vi "getWindowSnapshot.vi"(8 "error in (no error)":errorcluster, 11 "Registered Name":string) -> (0 "error out":errorcluster, 3 "Cropped Image Data":T1)   [LabVIEW 2018, in "Image_Diff.lvlib"]
uses:
  Image_Diff.lvlib
  <vilib>/picture/picture.llb/imagedata.ctl
panel:
  out "Cropped Picture":picture
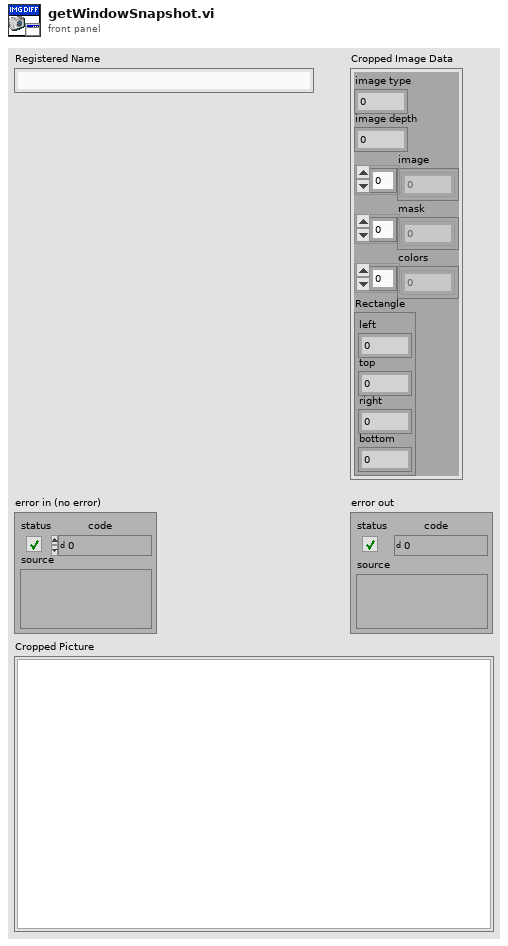
[diagram p1: front panel]
types:
  T1 = typedef "imagedata.ctl" = cluster{"image type":i32, "image depth":i32, "image":u8[], "mask":u8[], "colors":u32[], "Rectangle":cluster{"left":i16, "top":i16, "right":i16, "bottom":i16}}
  T2 = cluster{"left":i32, "top":i32, "right":i32, "bottom":i32}
  T3 = enum32{"Invalid", "Standard", "Closed", "Hidden", "Minimized", "Maximized"}
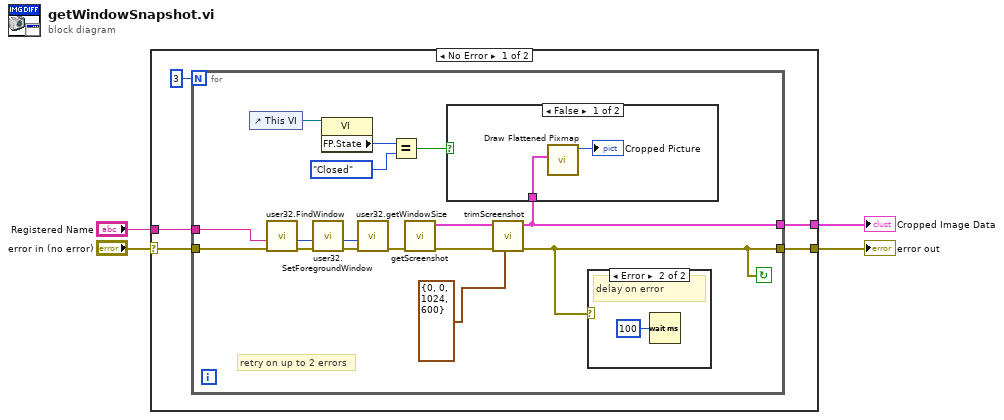
[diagram p0: block diagram]
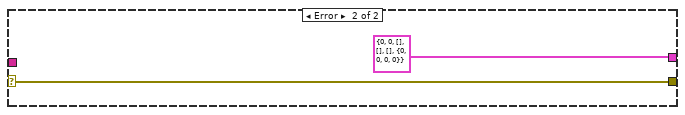
[diagram p4: hidden frame]
diagram:
  n1 = case shown="No Error" "error in (no error)" {
    selector: "error in (no error)" -> [w9 w29]
    tunnel: "Registered Name" -> [w6 _]
    tunnel: [w8 w29] -> w2
    tunnel: [w7 T1 {"image type"=0, "image depth"=0, "image"=[], "mask"=[], "colors"=[], "Rectangle"={"left"=0, "top"=0, "right"=0, "bottom"=0}} ("Cropped Image Data")] -> w1
    frame No Error {
      n2 = for {
        N: 3 -> [_]
        tunnel: [w13] -> w7
        tunnel: w6 -> [w12]
        tunnel: w9 -> [w21]
        tunnel: [w10] -> w8
        stop <- w10 continue-if-true
        # "retry on up to 2 errors"
        n3 = control-ref of="This VI"() -> (w17:refnum<vi>)
        n4 = call "user32.FindWindow.vi"("error in"=w21, "Window Title"=w12) -> ("error out"=w25:errorcluster, "hWnd"=w23:u32)  [unwired: 8 in]
        n5 = call "user32.SetForegroundWindow.vi"("error in"=w25, "hWnd"=w23) -> ("error out"=w24:errorcluster, "hWnd out"=w22:u32)  [unwired: 8 in]
        n6 = property class="VI"(reference=w17) -> ("FP.State"=w16:T3)  [unwired: 1 in, 2 out]
        n7 = call "user32.getWindowSize.vi"("error in"=w24, "hWnd"=w22) -> ("error out"=w20:errorcluster)  [unwired: 7 in, 2 out]
        n8 = Equal?(x=w16, y=T3."Closed") -> (x = y?=w14:bool)
        n9 = call "getScreenshot.vi"("error in (no error)"=w20) -> ("error out"=w18:errorcluster, "Image Data"=w19:T1)  [unwired: 9 in]
        n10 = call "trimScreenshot.vi"("Crop Rectangle"=T2 {"left"=0, "top"=0, "right"=1024, "bottom"=600} ("Rectangle Coordinates"), "error in (no error)"=w18, "Flattened Image Data"=w19) -> ("error out"=w10:errorcluster, "Cropped Image Data"=w13:T1)  [unwired: 7 in]
        n11 = case shown="False" w14 {
          tunnel: w13 -> [w28 _]
          frame False {
            n12 = call <vilib>:"Draw Flattened Pixmap.vi"("image data"=w28) -> ("new picture"=→"Cropped Picture":picture)  [unwired: 8 in]
          }
          frame True {
          }
        }
        n13 = case shown="Error" w10 {
          frame No Error {
          }
          frame Error {
            # "delay on error"
            n14 = Wait (ms)(milliseconds to wait=u32 100) -> ()  [unwired: 1 out]
          }
        }
      }
    }
    frame Error {
    }
  }
  "error out" <- w2
  "Cropped Image Data" <- w1
